vi "Dual_Motor.vi"(5 "refnum name 2":string="My Motor RefNum", 7 "refnum name 1":string="My Motor RefNum", 8 "Back speed":dbl, 9 "For Speed":dbl, 10 "Backward":bool, 11 "Forward":bool) -> ()   [LabVIEW 2017]
panel:
  in  "Reverse?":bool
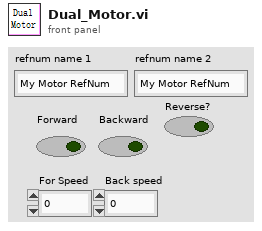
[diagram p1: front panel]
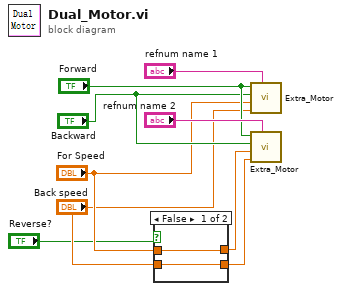
[diagram p0: block diagram]
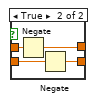
[diagram p2: hidden frame]
diagram:
  n1 = case shown="False" "Reverse?" {
    tunnel: "For Speed" -> [w11 w15]
    tunnel: "Back speed" -> [w10 w14]
    tunnel: [w11 w13] -> w3
    tunnel: [w10 w12] -> w2
    frame False {
    }
    frame True {
      n2 = Negate(x=w15) -> (-x=w13:dbl)
      n3 = Negate(x=w14) -> (-x=w12:dbl)
    }
  }
  n4 = call "Extra_Motor.vi"("refnum name"="refnum name 1", "Back Speed"="Back speed", "For Speed"="For Speed", "Backward"="Backward", "Forward"="Forward") -> ()  [unwired: 7 in]
  n5 = call "Extra_Motor.vi"("refnum name"="refnum name 2", "Back Speed"=w2, "For Speed"=w3, "Backward"="Backward", "Forward"="Forward") -> ()  [unwired: 7 in]
